vi "Get frf variation.vi"(9 "# taps / position":i32=1, 11 "Files":path[](array[path])=[path "/Users/crogers/Dropbox (Rogers)/Violin Stuff/PC ViolnData/SoundCard2/SoundCard2 ModalShop7/Raw/SoundCard2 ModalShop7 H_001_001.wfm", path "/Users/crogers/Dropbox (Rogers)/Violin Stuff/PC ViolnData/SoundCard2/SoundCard2 ModalShop7/Raw/SoundCard2 ModalShop7 H_001_002.wfm", path "/Users/crogers/Dropbox (Rogers)/Violin Stuff/PC ViolnData/SoundCard2/SoundCard2 ModalShop7/Raw/SoundCard2 ModalShop7 H_001_003.wfm", path "/Users/crogers/Dropbox (Rogers)/Violin Stuff/PC ViolnData/SoundCard2/SoundCard2 ModalShop7/Raw/SoundCard2 ModalShop7 H_001_004.wfm", path "/Users/crogers/Dropbox (Rogers)/Violin Stuff/PC ViolnData/SoundCard2/SoundCard2 ModalShop7/Raw/SoundCard2 ModalShop7 H_001_005.wfm", path "/Users/crogers/Dropbox (Rogers)/Violin Stuff/PC ViolnData/SoundCard2/SoundCard2 ModalShop7/Raw/SoundCard2 ModalShop7 H_001_006.wfm", path "/Users/crogers/Dropbox (Rogers)/Violin Stuff/PC ViolnData/SoundCard2/SoundCard2 ModalShop7/Raw/SoundCard2 ModalShop7 H_001_007.wfm", path "/Users/crogers/Dropbox (Rogers)/Violin Stuff/PC ViolnData/SoundCard2/SoundCard2 ModalShop7/Raw/SoundCard2 ModalShop7 H_001_008.wfm", path "/Users/crogers/Dropbox (Rogers)/Violin Stuff/PC ViolnData/SoundCard2/SoundCard2 ModalShop7/Raw/SoundCard2 ModalShop7 H_001_009.wfm", path "/Users/crogers/Dropbox (Rogers)/Violin Stuff/PC ViolnData/SoundCard2/SoundCard2 ModalShop7/Raw/SoundCard2 ModalShop7 H_001_010.wfm", path "/Users/crogers/Dropbox (Rogers)/Violin Stuff/PC ViolnData/SoundCard2/SoundCard2 ModalShop7/Raw/SoundCard2 ModalShop7 H_002_001.wfm", path "/Users/crogers/Dropbox (Rogers)/Violin Stuff/PC ViolnData/SoundCard2/SoundCard2 ModalShop7/Raw/SoundCard2 ModalShop7 H_002_002.wfm", path "/Users/crogers/Dropbox (Rogers)/Violin Stuff/PC ViolnData/SoundCard2/SoundCard2 ModalShop7/Raw/SoundCard2 ModalShop7 H_002_003.wfm", path "/Users/crogers/Dropbox (Rogers)/Violin Stuff/PC ViolnData/SoundCard2/SoundCard2 ModalShop7/Raw/SoundCard2 ModalShop7 H_002_004.wfm", path "/Users/crogers/Dropbox (Rogers)/Violin Stuff/PC ViolnData/SoundCard2/SoundCard2 ModalShop7/Raw/SoundCard2 ModalShop7 H_002_005.wfm", path "/Users/crogers/Dropbox (Rogers)/Violin Stuff/PC ViolnData/SoundCard2/SoundCard2 ModalShop7/Raw/SoundCard2 ModalShop7 H_002_006.wfm", path "/Users/crogers/Dropbox (Rogers)/Violin Stuff/PC ViolnData/SoundCard2/SoundCard2 ModalShop7/Raw/SoundCard2 ModalShop7 H_002_007.wfm", path "/Users/crogers/Dropbox (Rogers)/Violin Stuff/PC ViolnData/SoundCard2/SoundCard2 ModalShop7/Raw/SoundCard2 ModalShop7 H_002_008.wfm", path "/Users/crogers/Dropbox (Rogers)/Violin Stuff/PC ViolnData/SoundCard2/SoundCard2 ModalShop7/Raw/SoundCard2 ModalShop7 H_002_009.wfm", path "/Users/crogers/Dropbox (Rogers)/Violin Stuff/PC ViolnData/SoundCard2/SoundCard2 ModalShop7/Raw/SoundCard2 ModalShop7 H_002_010.wfm", path "/Users/crogers/Dropbox (Rogers)/Violin Stuff/PC ViolnData/SoundCard2/SoundCard2 ModalShop7/Raw/SoundCard2 ModalShop7 H_003_001.wfm", path "/Users/crogers/Dropbox (Rogers)/Violin Stuff/PC ViolnData/SoundCard2/SoundCard2 ModalShop7/Raw/SoundCard2 ModalShop7 H_003_002.wfm", path "/Users/crogers/Dropbox (Rogers)/Violin Stuff/PC ViolnData/SoundCard2/SoundCard2 ModalShop7/Raw/SoundCard2 ModalShop7 H_003_003.wfm", path "/Users/crogers/Dropbox (Rogers)/Violin Stuff/PC ViolnData/SoundCard2/SoundCard2 ModalShop7/Raw/SoundCard2 ModalShop7 H_003_004.wfm", path "/Users/crogers/Dropbox (Rogers)/Violin Stuff/PC ViolnData/SoundCard2/SoundCard2 ModalShop7/Raw/SoundCard2 ModalShop7 H_003_005.wfm", path "/Users/crogers/Dropbox (Rogers)/Violin Stuff/PC ViolnData/SoundCard2/SoundCard2 ModalShop7/Raw/SoundCard2 ModalShop7 H_003_006.wfm", path "/Users/crogers/Dropbox (Rogers)/Violin Stuff/PC ViolnData/SoundCard2/SoundCard2 ModalShop7/Raw/SoundCard2 ModalShop7 H_003_007.wfm", path "/Users/crogers/Dropbox (Rogers)/Violin Stuff/PC ViolnData/SoundCard2/SoundCard2 ModalShop7/Raw/SoundCard2 ModalShop7 H_003_008.wfm", path "/Users/crogers/Dropbox (Rogers)/Violin Stuff/PC ViolnData/SoundCard2/SoundCard2 ModalShop7/Raw/SoundCard2 ModalShop7 H_003_009.wfm", path "/Users/crogers/Dropbox (Rogers)/Violin Stuff/PC ViolnData/SoundCard2/SoundCard2 ModalShop7/Raw/SoundCard2 ModalShop7 H_003_010.wfm", path "/Users/crogers/Dropbox (Rogers)/Violin Stuff/PC ViolnData/SoundCard2/SoundCard2 ModalShop7/Raw/SoundCard2 ModalShop7 H_004_001.wfm", path "/Users/crogers/Dropbox (Rogers)/Violin Stuff/PC ViolnData/SoundCard2/SoundCard2 ModalShop7/Raw/SoundCard2 ModalShop7 H_004_002.wfm", path "/Users/crogers/Dropbox (Rogers)/Violin Stuff/PC ViolnData/SoundCard2/SoundCard2 ModalShop7/Raw/SoundCard2 ModalShop7 H_004_003.wfm", path "/Users/crogers/Dropbox (Rogers)/Violin Stuff/PC ViolnData/SoundCard2/SoundCard2 ModalShop7/Raw/SoundCard2 ModalShop7 H_004_004.wfm", path "/Users/crogers/Dropbox (Rogers)/Violin Stuff/PC ViolnData/SoundCard2/SoundCard2 ModalShop7/Raw/SoundCard2 ModalShop7 H_004_005.wfm", path "/Users/crogers/Dropbox (Rogers)/Violin Stuff/PC ViolnData/SoundCard2/SoundCard2 ModalShop7/Raw/SoundCard2 ModalShop7 H_004_006.wfm", path "/Users/crogers/Dropbox (Rogers)/Violin Stuff/PC ViolnData/SoundCard2/SoundCard2 ModalShop7/Raw/SoundCard2 ModalShop7 H_004_007.wfm", path "/Users/crogers/Dropbox (Rogers)/Violin Stuff/PC ViolnData/SoundCard2/SoundCard2 ModalShop7/Raw/SoundCard2 ModalShop7 H_004_008.wfm", path "/Users/crogers/Dropbox (Rogers)/Violin Stuff/PC ViolnData/SoundCard2/SoundCard2 ModalShop7/Raw/SoundCard2 ModalShop7 H_004_009.wfm", path "/Users/crogers/Dropbox (Rogers)/Violin Stuff/PC ViolnData/SoundCard2/SoundCard2 ModalShop7/Raw/SoundCard2 ModalShop7 H_004_010.wfm", path "/Users/crogers/Dropbox (Rogers)/Violin Stuff/PC ViolnData/SoundCard2/SoundCard2 ModalShop7/Raw/SoundCard2 ModalShop7 H_005_001.wfm", path "/Users/crogers/Dropbox (Rogers)/Violin Stuff/PC ViolnData/SoundCard2/SoundCard2 ModalShop7/Raw/SoundCard2 ModalShop7 H_005_002.wfm", path "/Users/crogers/Dropbox (Rogers)/Violin Stuff/PC ViolnData/SoundCard2/SoundCard2 ModalShop7/Raw/SoundCard2 ModalShop7 H_005_003.wfm", path "/Users/crogers/Dropbox (Rogers)/Violin Stuff/PC ViolnData/SoundCard2/SoundCard2 ModalShop7/Raw/SoundCard2 ModalShop7 H_005_004.wfm", path "/Users/crogers/Dropbox (Rogers)/Violin Stuff/PC ViolnData/SoundCard2/SoundCard2 ModalShop7/Raw/SoundCard2 ModalShop7 H_005_005.wfm", path "/Users/crogers/Dropbox (Rogers)/Violin Stuff/PC ViolnData/SoundCard2/SoundCard2 ModalShop7/Raw/SoundCard2 ModalShop7 H_005_006.wfm", path "/Users/crogers/Dropbox (Rogers)/Violin Stuff/PC ViolnData/SoundCard2/SoundCard2 ModalShop7/Raw/SoundCard2 ModalShop7 H_005_007.wfm", path "/Users/crogers/Dropbox (Rogers)/Violin Stuff/PC ViolnData/SoundCard2/SoundCard2 ModalShop7/Raw/SoundCard2 ModalShop7 H_005_008.wfm", path "/Users/crogers/Dropbox (Rogers)/Violin Stuff/PC ViolnData/SoundCard2/SoundCard2 ModalShop7/Raw/SoundCard2 ModalShop7 H_005_009.wfm", path "/Users/crogers/Dropbox (Rogers)/Violin Stuff/PC ViolnData/SoundCard2/SoundCard2 ModalShop7/Raw/SoundCard2 ModalShop7 H_005_010.wfm", path "/Users/crogers/Dropbox (Rogers)/Violin Stuff/PC ViolnData/SoundCard2/SoundCard2 ModalShop8/Raw/SoundCard2 ModalShop8 H_001_001.wfm", path "/Users/crogers/Dropbox (Rogers)/Violin Stuff/PC ViolnData/SoundCard2/SoundCard2 ModalShop8/Raw/SoundCard2 ModalShop8 H_001_002.wfm", path "/Users/crogers/Dropbox (Rogers)/Violin Stuff/PC ViolnData/SoundCard2/SoundCard2 ModalShop8/Raw/SoundCard2 ModalShop8 H_001_003.wfm", path "/Users/crogers/Dropbox (Rogers)/Violin Stuff/PC ViolnData/SoundCard2/SoundCard2 ModalShop8/Raw/SoundCard2 ModalShop8 H_001_004.wfm", path "/Users/crogers/Dropbox (Rogers)/Violin Stuff/PC ViolnData/SoundCard2/SoundCard2 ModalShop8/Raw/SoundCard2 ModalShop8 H_001_005.wfm", path "/Users/crogers/Dropbox (Rogers)/Violin Stuff/PC ViolnData/SoundCard2/SoundCard2 ModalShop8/Raw/SoundCard2 ModalShop8 H_001_006.wfm", path "/Users/crogers/Dropbox (Rogers)/Violin Stuff/PC ViolnData/SoundCard2/SoundCard2 ModalShop8/Raw/SoundCard2 ModalShop8 H_001_007.wfm", path "/Users/crogers/Dropbox (Rogers)/Violin Stuff/PC ViolnData/SoundCard2/SoundCard2 ModalShop8/Raw/SoundCard2 ModalShop8 H_001_008.wfm", path "/Users/crogers/Dropbox (Rogers)/Violin Stuff/PC ViolnData/SoundCard2/SoundCard2 ModalShop8/Raw/SoundCard2 ModalShop8 H_001_009.wfm", path "/Users/crogers/Dropbox (Rogers)/Violin Stuff/PC ViolnData/SoundCard2/SoundCard2 ModalShop8/Raw/SoundCard2 ModalShop8 H_001_010.wfm", path "/Users/crogers/Dropbox (Rogers)/Violin Stuff/PC ViolnData/SoundCard2/SoundCard2 ModalShop8/Raw/SoundCard2 ModalShop8 H_002_001.wfm", path "/Users/crogers/Dropbox (Rogers)/Violin Stuff/PC ViolnData/SoundCard2/SoundCard2 ModalShop8/Raw/SoundCard2 ModalShop8 H_002_002.wfm", path "/Users/crogers/Dropbox (Rogers)/Violin Stuff/PC ViolnData/SoundCard2/SoundCard2 ModalShop8/Raw/SoundCard2 ModalShop8 H_002_003.wfm", path "/Users/crogers/Dropbox (Rogers)/Violin Stuff/PC ViolnData/SoundCard2/SoundCard2 ModalShop8/Raw/SoundCard2 ModalShop8 H_002_004.wfm", path "/Users/crogers/Dropbox (Rogers)/Violin Stuff/PC ViolnData/SoundCard2/SoundCard2 ModalShop8/Raw/SoundCard2 ModalShop8 H_002_005.wfm", path "/Users/crogers/Dropbox (Rogers)/Violin Stuff/PC ViolnData/SoundCard2/SoundCard2 ModalShop8/Raw/SoundCard2 ModalShop8 H_002_006.wfm", path "/Users/crogers/Dropbox (Rogers)/Violin Stuff/PC ViolnData/SoundCard2/SoundCard2 ModalShop8/Raw/SoundCard2 ModalShop8 H_002_007.wfm", path "/Users/crogers/Dropbox (Rogers)/Violin Stuff/PC ViolnData/SoundCard2/SoundCard2 ModalShop8/Raw/SoundCard2 ModalShop8 H_002_008.wfm", path "/Users/crogers/Dropbox (Rogers)/Violin Stuff/PC ViolnData/SoundCard2/SoundCard2 ModalShop8/Raw/SoundCard2 ModalShop8 H_002_009.wfm", path "/Users/crogers/Dropbox (Rogers)/Violin Stuff/PC ViolnData/SoundCard2/SoundCard2 ModalShop8/Raw/SoundCard2 ModalShop8 H_002_010.wfm", path "/Users/crogers/Dropbox (Rogers)/Violin Stuff/PC ViolnData/SoundCard2/SoundCard2 ModalShop8/Raw/SoundCard2 ModalShop8 H_003_001.wfm", path "/Users/crogers/Dropbox (Rogers)/Violin Stuff/PC ViolnData/SoundCard2/SoundCard2 ModalShop8/Raw/SoundCard2 ModalShop8 H_003_002.wfm", path "/Users/crogers/Dropbox (Rogers)/Violin Stuff/PC ViolnData/SoundCard2/SoundCard2 ModalShop8/Raw/SoundCard2 ModalShop8 H_003_003.wfm", path "/Users/crogers/Dropbox (Rogers)/Violin Stuff/PC ViolnData/SoundCard2/SoundCard2 ModalShop8/Raw/SoundCard2 ModalShop8 H_003_004.wfm", path "/Users/crogers/Dropbox (Rogers)/Violin Stuff/PC ViolnData/SoundCard2/SoundCard2 ModalShop8/Raw/SoundCard2 ModalShop8 H_003_005.wfm", path "/Users/crogers/Dropbox (Rogers)/Violin Stuff/PC ViolnData/SoundCard2/SoundCard2 ModalShop8/Raw/SoundCard2 ModalShop8 H_003_006.wfm", path "/Users/crogers/Dropbox (Rogers)/Violin Stuff/PC ViolnData/SoundCard2/SoundCard2 ModalShop8/Raw/SoundCard2 ModalShop8 H_003_007.wfm", path "/Users/crogers/Dropbox (Rogers)/Violin Stuff/PC ViolnData/SoundCard2/SoundCard2 ModalShop8/Raw/SoundCard2 ModalShop8 H_003_008.wfm", path "/Users/crogers/Dropbox (Rogers)/Violin Stuff/PC ViolnData/SoundCard2/SoundCard2 ModalShop8/Raw/SoundCard2 ModalShop8 H_003_009.wfm", path "/Users/crogers/Dropbox (Rogers)/Violin Stuff/PC ViolnData/SoundCard2/SoundCard2 ModalShop8/Raw/SoundCard2 ModalShop8 H_003_010.wfm", path "/Users/crogers/Dropbox (Rogers)/Violin Stuff/PC ViolnData/SoundCard2/SoundCard2 ModalShop8/Raw/SoundCard2 ModalShop8 H_004_001.wfm", path "/Users/crogers/Dropbox (Rogers)/Violin Stuff/PC ViolnData/SoundCard2/SoundCard2 ModalShop8/Raw/SoundCard2 ModalShop8 H_004_002.wfm", path "/Users/crogers/Dropbox (Rogers)/Violin Stuff/PC ViolnData/SoundCard2/SoundCard2 ModalShop8/Raw/SoundCard2 ModalShop8 H_004_003.wfm", path "/Users/crogers/Dropbox (Rogers)/Violin Stuff/PC ViolnData/SoundCard2/SoundCard2 ModalShop8/Raw/SoundCard2 ModalShop8 H_004_004.wfm", path "/Users/crogers/Dropbox (Rogers)/Violin Stuff/PC ViolnData/SoundCard2/SoundCard2 ModalShop8/Raw/SoundCard2 ModalShop8 H_004_005.wfm", path "/Users/crogers/Dropbox (Rogers)/Violin Stuff/PC ViolnData/SoundCard2/SoundCard2 ModalShop8/Raw/SoundCard2 ModalShop8 H_004_006.wfm", path "/Users/crogers/Dropbox (Rogers)/Violin Stuff/PC ViolnData/SoundCard2/SoundCard2 ModalShop8/Raw/SoundCard2 ModalShop8 H_004_007.wfm", path "/Users/crogers/Dropbox (Rogers)/Violin Stuff/PC ViolnData/SoundCard2/SoundCard2 ModalShop8/Raw/SoundCard2 ModalShop8 H_004_008.wfm", path "/Users/crogers/Dropbox (Rogers)/Violin Stuff/PC ViolnData/SoundCard2/SoundCard2 ModalShop8/Raw/SoundCard2 ModalShop8 H_004_009.wfm", path "/Users/crogers/Dropbox (Rogers)/Violin Stuff/PC ViolnData/SoundCard2/SoundCard2 ModalShop8/Raw/SoundCard2 ModalShop8 H_004_010.wfm", path "/Users/crogers/Dropbox (Rogers)/Violin Stuff/PC ViolnData/SoundCard2/SoundCard2 ModalShop8/Raw/SoundCard2 ModalShop8 H_005_001.wfm", path "/Users/crogers/Dropbox (Rogers)/Violin Stuff/PC ViolnData/SoundCard2/SoundCard2 ModalShop8/Raw/SoundCard2 ModalShop8 H_005_002.wfm", path "/Users/crogers/Dropbox (Rogers)/Violin Stuff/PC ViolnData/SoundCard2/SoundCard2 ModalShop8/Raw/SoundCard2 ModalShop8 H_005_003.wfm", path "/Users/crogers/Dropbox (Rogers)/Violin Stuff/PC ViolnData/SoundCard2/SoundCard2 ModalShop8/Raw/SoundCard2 ModalShop8 H_005_004.wfm", path "/Users/crogers/Dropbox (Rogers)/Violin Stuff/PC ViolnData/SoundCard2/SoundCard2 ModalShop8/Raw/SoundCard2 ModalShop8 H_005_005.wfm", path "/Users/crogers/Dropbox (Rogers)/Violin Stuff/PC ViolnData/SoundCard2/SoundCard2 ModalShop8/Raw/SoundCard2 ModalShop8 H_005_006.wfm", path "/Users/crogers/Dropbox (Rogers)/Violin Stuff/PC ViolnData/SoundCard2/SoundCard2 ModalShop8/Raw/SoundCard2 ModalShop8 H_005_007.wfm", path "/Users/crogers/Dropbox (Rogers)/Violin Stuff/PC ViolnData/SoundCard2/SoundCard2 ModalShop8/Raw/SoundCard2 ModalShop8 H_005_008.wfm", path "/Users/crogers/Dropbox (Rogers)/Violin Stuff/PC ViolnData/SoundCard2/SoundCard2 ModalShop8/Raw/SoundCard2 ModalShop8 H_005_009.wfm", path "/Users/crogers/Dropbox (Rogers)/Violin Stuff/PC ViolnData/SoundCard2/SoundCard2 ModalShop8/Raw/SoundCard2 ModalShop8 H_005_010.wfm"]) -> (2 "sdev":dbl[](array[numeric]), 3 "mean":dbl[](array[numeric]))   [LabVIEW 2024]
uses:
  PreferencesControl.ctl
  <vilib>/Analysis/NI_AALBase.lvlib
  <vilib>/Analysis/NI_AALPro.lvlib
panel:
  in  "Color Table":T1(ring)=enum."Rainbow-striped"
  out "Intensity Graph":i32[][](graph)
  out "ampl 2":dbl[](graph)
  out "Histogram Graph":T2(graph)
  out "ampl":dbl[](graph)
  out "Hammer Spectra":cluster{dbl, "df":dbl, "FFT {X}":dbl[]}[](graph)=[{0.0, "df"=1.0, "FFT {X}"=array[24001 elements]}]
  out "Microphone Spectra":cluster{"x0":dbl, "df":dbl, dbl[]}[](graph)=[{"x0"=0.0, "df"=1.0, array[24001 elements]}]
  out "Average FRF":cluster{dbl, "df":dbl, dbl[]}[](graph)=[{0.0, "df"=1.0, array[24001 elements]}, {0.0, "df"=1.0, array[24001 elements]}]
  out "Hammer":cluster{dbl, "dt":dbl, "Y":dbl[]}[](graph)=[{0.0, "dt"=2.0833333333333333e-05, "Y"=array[14400 elements]}]
  out "Microphone":cluster{dbl, "dt":dbl, "Y":dbl[]}[](graph)=[{0.0, "dt"=2.0833333333333333e-05, "Y"=array[14400 elements]}]
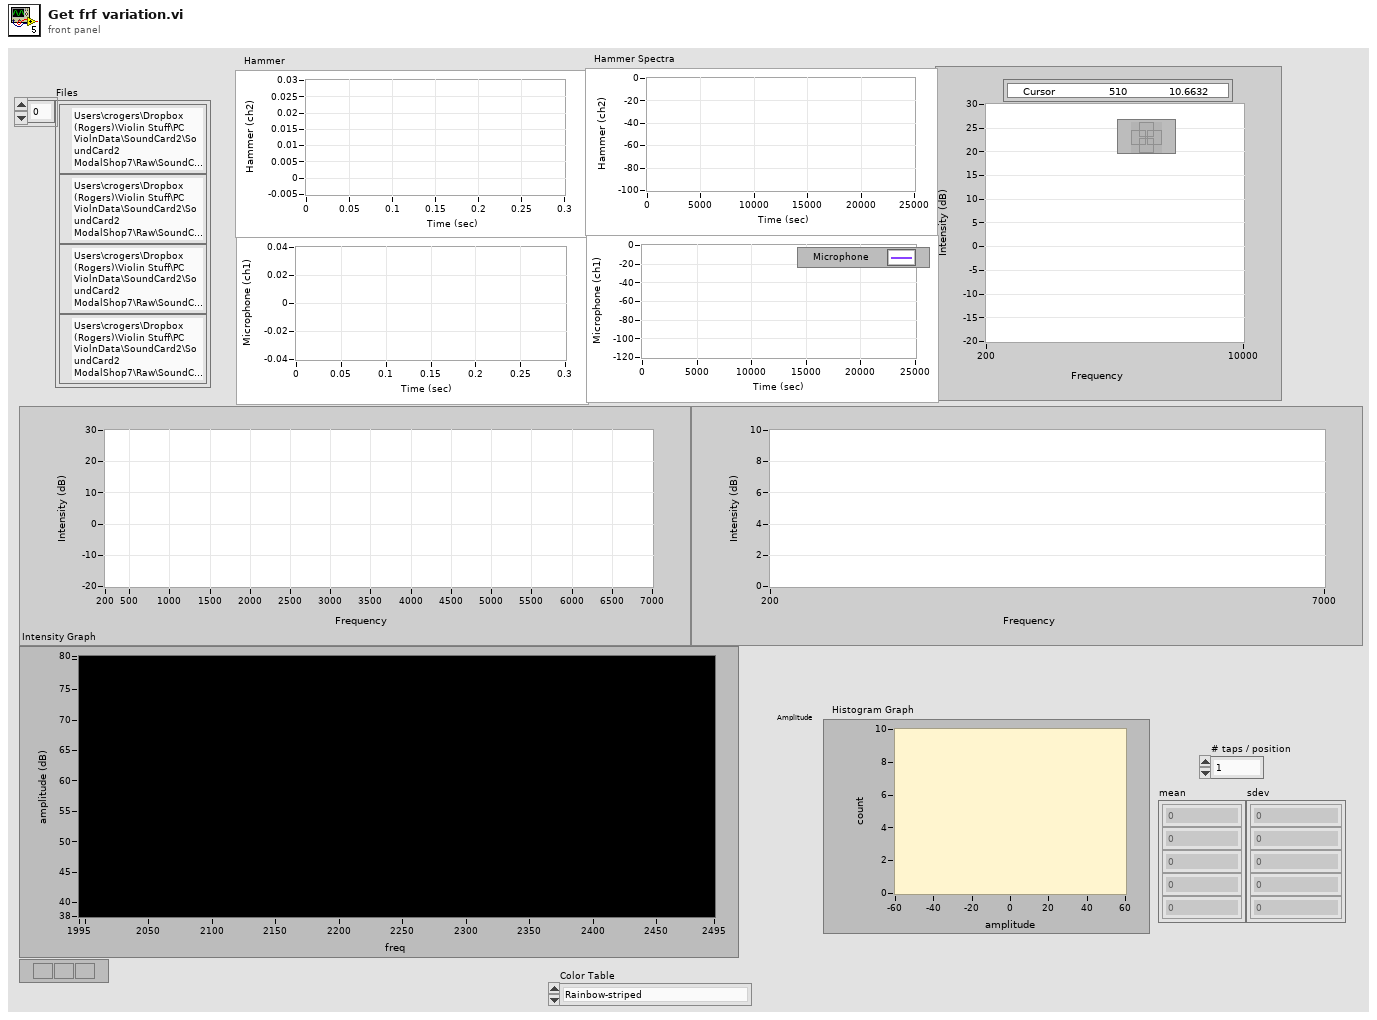
[diagram p1: front panel]
types:
  T1 = enum16{"Apricot", "Carnation", "Ether", "Greyscale", "Greyscale-banded", "Hot Metal", "Lava Waves", "Mac", "Morning Glory", "Rainbow", "Rainbow-banded", "Rainbow-inverted", "Rainbow-striped", "Saturn", "Seismic", "Space"}
  T2 = cluster{"X Values":dbl[], "Histogram: h(x)":i32[]}[]
  T3 = typedef "PreferencesControl.ctl" = cluster{"Name of test":string, "Date":timestamp, "Location":string, "Template":string, "Soundcard":string, "resolution":u16, "Sampling rate":u16, "Ch1 Gain ":dbl, "Ch2 Gain":dbl, "Sample time (s)":dbl, "Pre-trigger (s)":dbl, "Hammer Threshold":dbl, "Positions":i16, "Taps/Position":i16, "Set Names":string, "Freq resolution":dbl, "Hammer cutoff":dbl, "Mic cutoff":dbl, "Double bounce ":dbl, "Hammer Cal":dbl, "dB Offset":dbl, "Accel Cal":dbl, "Vibrometer Cal":dbl, "Mic Cal":dbl, "Output":u16, "Voltage Cal":dbl, "Vibrometer Port":refnum<visa-resource-name>, "Range":u16, "High Pass":u16, "Bandwidth":u16, "X Range":cluster{"Minimum":dbl, "Maximum":dbl, "Increment":dbl, "Minor Increment":dbl, "Start":dbl}[], "Y Range":cluster{"Minimum":dbl, "Maximum":dbl, "Increment":dbl, "Minor Increment":dbl, "Start":dbl}[], "dB Spread":dbl, "Trigger":u16, "Ch_1":u8, "Ch_2":u8, "flip?":bool, "60Hz":bool, "Time offset":dbl, "Piezo Cal":dbl, "Default Notes":string}
  T4 = cluster{"lower":dbl, "upper":dbl, "inclusion":enum32{"lower", "upper", "both", "neither"}}
  T5 = cluster{"X Values":dbl[], "Histogram: h(x)":i32[]}
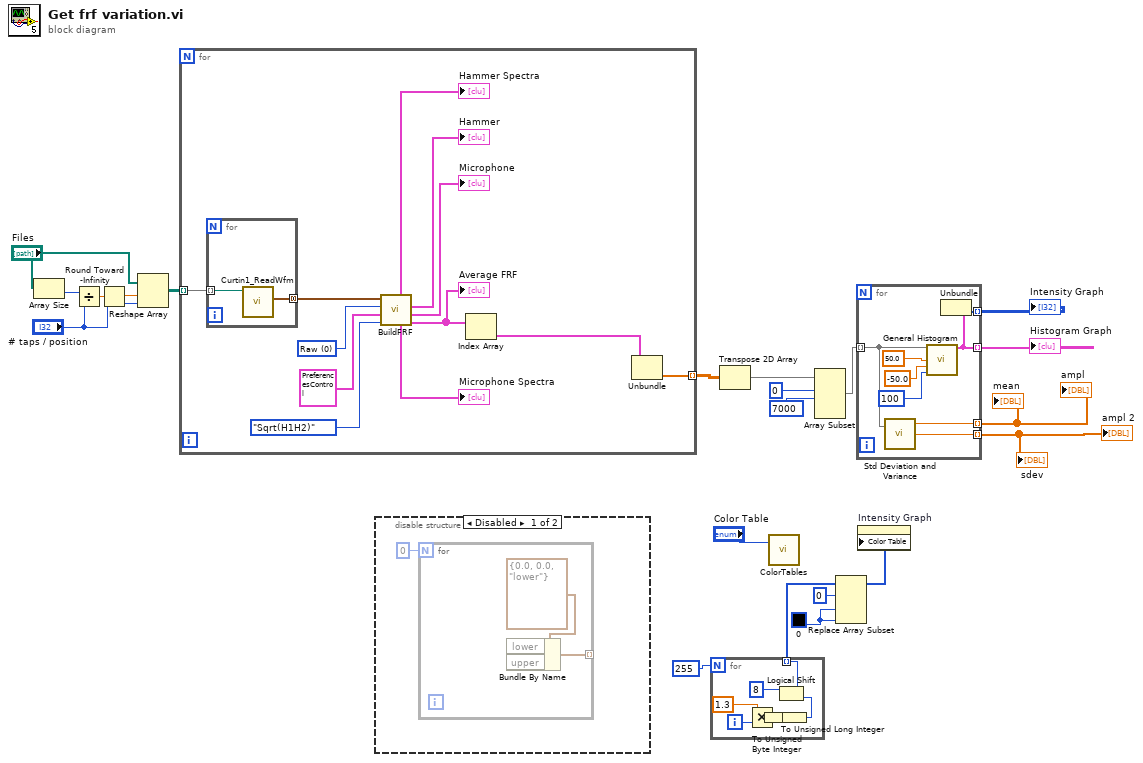
[diagram p0: block diagram]
diagram:
  w3 = u32 0
  n1 = Array Size(array="Files") -> (size(s)=w18:i32)
  n2 = Divide(x=w18, y="# taps / position") -> (x/y=w16:dbl)
  n3 = Round Toward -Infinity(1:w16) -> (0:w13:dbl)
  n4 = Reshape Array("Files", w13, "# taps / position") -> (w21:path[][])
  n5 = for {
    tunnel: w21 -> [w24] mode=indexing
    tunnel: [w23] -> w20 mode=indexing
    w32 = u16 0 items=["Raw", "Volts", "Units (Pa, N, mm/s etc)"] ("View")
    n6 = for {
      tunnel: [w35] -> w33 mode=concatenating
      tunnel: w24 -> [w34] mode=indexing
      n7 = call "Curtin1_ReadWfm.vi"("appended path"=w34) -> ("all waveforms in record"=w35:waveform(dbl)[])  [unwired: 9 in, 1 out]
    }
    n8 = call "BuildFRF.vi"("Method"=enum16{"Sqrt(H1H2)", "H1", "H2"}."Sqrt(H1H2)", "Settings"=T3 {"Name of test"="SoundCard2--SoundCard2 Focusrite", "Date"=timestamp(3723372723 s since 1904-01-01), "Location"="Home", "Template"="ScratchPad", "Soundcard"="Microphone (Scarlett 2i2 USB)", "resolution"=32, "Sampling rate"=48000, "Ch1 Gain "=0.0, "Ch2 Gain"=0.0, "Sample time (s)"=0.3, "Pre-trigger (s)"=0.001, "Hammer Threshold"=0.3327868852459017, "Positions"=1, "Taps/Position"=20, "Set Names"="H", "Freq resolution"=1.0, "Hammer cutoff"=0.0056410256410256415, "Mic cutoff"=0.25, "Double bounce "=0.01, "Hammer Cal"=1.0, "dB Offset"=0.0, "Accel Cal"=1.0, "Vibrometer Cal"=1.0, "Mic Cal"=1.0, "Output"=2, "Voltage Cal"=1.0, "Vibrometer Port"="ASRL27::INSTR", "Range"=20, "High Pass"=0, "Bandwidth"=25, "X Range"=[{"Minimum"=200.0, "Maximum"=10000.0, "Increment"=10.0, "Minor Increment"=100.0, "Start"=200.0}, {"Minimum"=0.0, "Maximum"=0.05, "Increment"=0.025, "Minor Increment"=0.0025, "Start"=0.0}, {"Minimum"=-0.02, "Maximum"=0.3, "Increment"=0.1, "Minor Increment"=0.01, "Start"=0.0}, {"Minimum"=150.0, "Maximum"=10000.0, "Increment"=10.0, "Minor Increment"=100.0, "Start"=1000.0}], "Y Range"=[{"Minimum"=-25.0, "Maximum"=0.0, "Increment"=5.0, "Minor Increment"=1.0, "Start"=-25.0}, {"Minimum"=-0.1, "Maximum"=1.0, "Increment"=0.25, "Minor Increment"=0.05, "Start"=0.0}, {"Minimum"=-1.0, "Maximum"=1.0, "Increment"=0.5, "Minor Increment"=0.1, "Start"=-1.0}, {"Minimum"=-12.0, "Maximum"=28.0, "Increment"=1.0, "Minor Increment"=0.25, "Start"=-12.0}], "dB Spread"=40.0, "Trigger"=0, "Ch_1"=1, "Ch_2"=2, "flip?"=FALSE, "60Hz"=FALSE, "Time offset"=0.0, "Piezo Cal"=1.0, "Default Notes"=""}, "View"=w32, "Data In"=w33) -> ("Average FRF"=w25:cluster{dbl, "df":dbl, dbl[]}[], "Microphone"=→"Microphone":cluster{dbl, "dt":dbl, "Y":dbl[]}[], "Hammer"=→"Hammer":cluster{dbl, "dt":dbl, "Y":dbl[]}[], "Microphone Spectra"=→"Microphone Spectra":cluster{"x0":dbl, "df":dbl, dbl[]}[], "Hammer Spectra"=→"Hammer Spectra":cluster{dbl, "df":dbl, "FFT {X}":dbl[]}[])  [unwired: 2 in, 1 out]
    "Average FRF" <- w25
    n9 = Index Array(array=w25) -> (element=w22:cluster{dbl, "df":dbl, dbl[]})  [unwired: 1 in]
    n10 = Unbundle(w22) -> (w23:dbl[])  [unwired: 2 out]
  }
  n11 = disable-structure shown="Disabled" {
    frame Disabled {
      n12 = for {
        N: 0 -> [_]
        tunnel: [w37] -> _ mode=indexing
        n13 = Bundle By Name(cluster=T4 {"lower"=0.0, "upper"=0.0, "inclusion"=enum."lower"}) -> (w37:T4)  [unwired: 2 in]
      }
    }
    frame Enabled {
    }
  }
  n14 = for {
    N: 255 -> [_]
    tunnel: [w41] -> w1 mode=indexing
    i -> [w45]
    n15 = Multiply(x=1.3, y=w45) -> (x*y=w43:dbl)
    n16 = To Unsigned Byte Integer(number=w43) -> (unsigned 8bit integer=w39:u8)
    n17 = To Unsigned Long Integer(number=w39) -> (unsigned 32bit integer=w42:u32)
    n18 = Logical Shift(y=i16 8, x=w42) -> (x << y=w41:u32)
  }
  n19 = Transpose 2D Array(2D array=w20) -> (transposed array=w15:dbl[][])
  n20 = call "ColorTables.vi"("Color Table"="Color Table") -> ()  [unwired: 2 in, 1 out]
  n21 = Array Subset(array=w15, index (row)=0 ("index"), length (row)=7000 ("index")) -> (w10:dbl[][])  [unwired: 2 in]
  n22 = Replace Array Subset(array=w1, new element #1=w3, index #1=0 ("index"), new element #2=w3) -> (w4:u32[])  [unwired: 1 in]
  n23 = for {
    tunnel: w10 -> [w53] mode=indexing
    tunnel: [w47] -> w14 mode=indexing
    tunnel: [w52] -> w12 mode=indexing
    tunnel: [w51] -> w11 mode=indexing
    tunnel: [w46] -> w7 mode=indexing
    n24 = call <vilib>:"Std Deviation and Variance.vi"("X"=w53) -> ("mean"=w52:dbl, "standard deviation"=w51:dbl)  [unwired: 1 in, 1 out]
    n25 = call <vilib>:"General Histogram.vi"("X"=w53, "max"=50.0, "min"=-50.0, "# bins"=100) -> ("Histogram Graph"=w47:T5)  [unwired: 7 in, 4 out]
    n26 = Unbundle(w47) -> ("Histogram: h(x)"=w46:i32[])  [unwired: 1 out]
  }
  "ampl" <- w12
  "Histogram Graph" <- w14
  "mean" <- w12
  "sdev" <- w11
  "ampl 2" <- w11
  "Intensity Graph" <- w7
  n27 = property on="Intensity Graph" class="IntGraph (strict)"("Color Table"=w4) -> ()  [unwired: 2 in, 2 out]
